vi "AVS_Deactivate.vi"(0 "a_hHandle":i32) -> (4 "Output Value":i32)   [LabVIEW 2020]
uses:
  AvaSpecX64-DLL_9.4/avaspecx64.dll
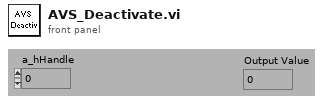
[diagram p1: front panel]
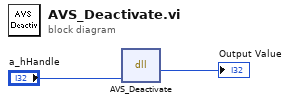
[diagram p0: block diagram]
diagram:
  n1 = dll-call lib="C:/AvaSpecX64-DLL_9.4/avaspecx64.dll" fn="AVS_Deactivate"("a_hHandle"="a_hHandle") -> ("return type"=→"Output Value":i32)  [unwired: 4 in, 2 out]
